vi "PI-C867-Joystick.vi"() -> ()   [LabVIEW 2026]
doc: "Demonstrates the fundamentals of the State Machine design pattern in LabVIEW. A state machine, in its simplest form, is a case structure within a while loop, with a state enum wired to a shift register on the loop to define the execution of different cases (or \"states\") of the case structure on different iterations of the loop."
uses:
  States.ctl
panel:
  out "WAIT":bool
  out "JoystickID":i32=3
  out "C687 Axes":string[](array[string])
  out "C687 System No.":i32=2
  out "Current positions":dbl[](array[numeric])=[0.0, -0.0002] format="%.6f"
  in  "Velocity array":dbl[](array[numeric])=[0.05, 0.1, 0.25, 0.5, 1.0, 10.0]
  in  "Joystick":bool
  out "Current velocity":dbl[](array[numeric])=[10.0, 10.0] format="%.6f"
  in  "Stop":bool
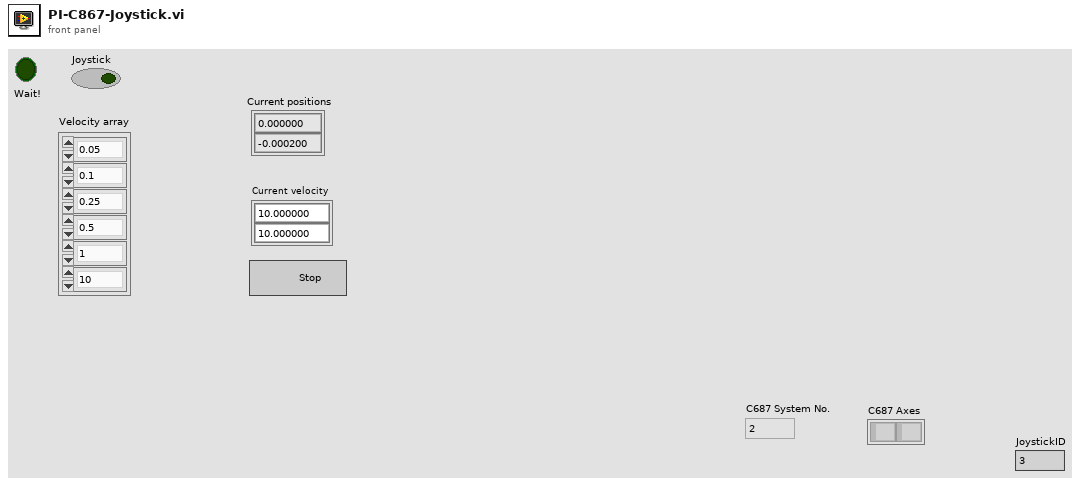
[diagram p1: front panel]
types:
  T1 = typedef "States.ctl" = enum16{"Initialize", "Wait for Event", "Joystick ON/OFF", "Button Pressed", "Stop"}
  T2 = cluster{"C687 System No.":i32, "JoystickID to query":i32[], "Conn.  Axes":string[], "State":bool[][], "Current velocity":dbl[], "Current positions":dbl[]}
  T3 = cluster{"RON Affected axes":string[], "Reference mode":bool[], "Check FRF?":bool}
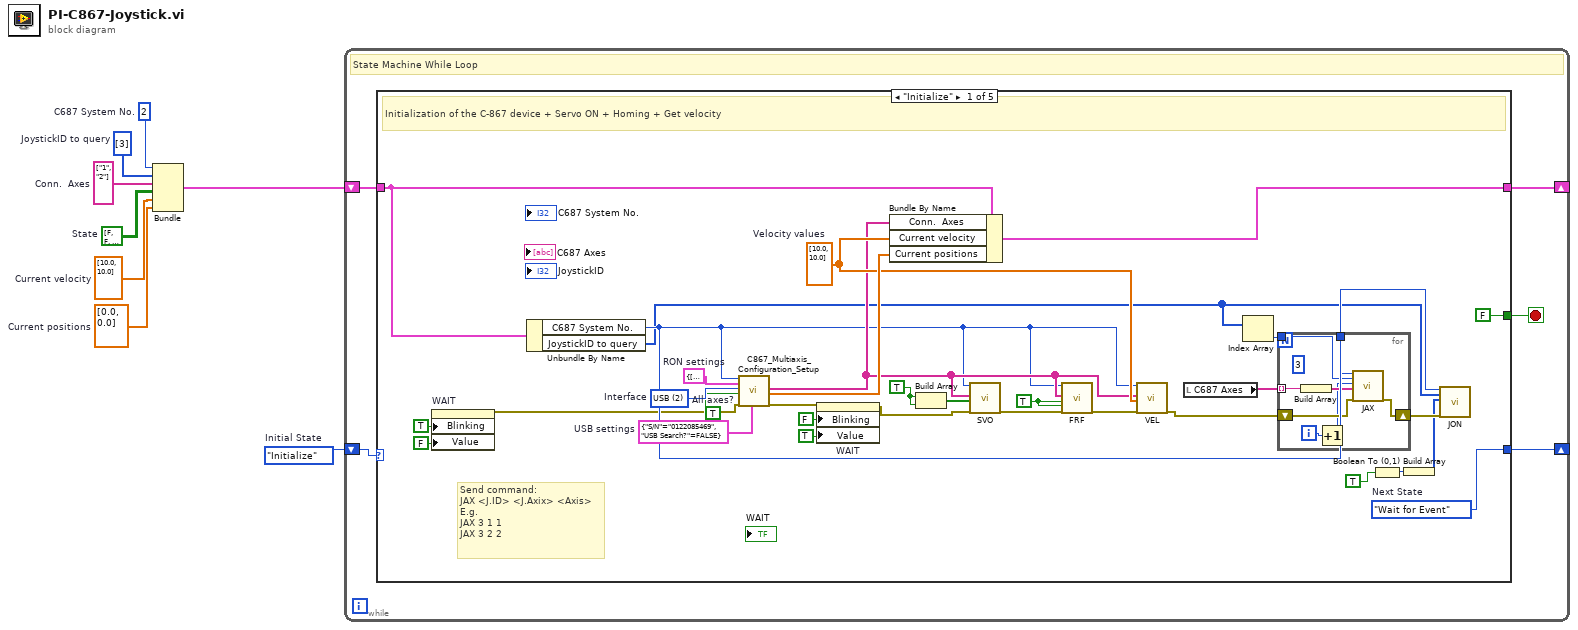
[diagram p0: block diagram]
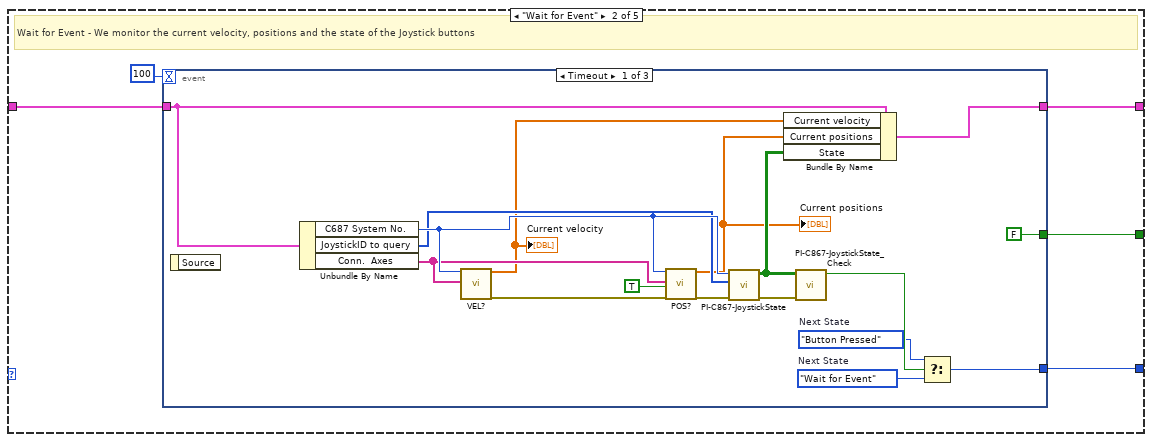
[diagram p2: hidden frame]
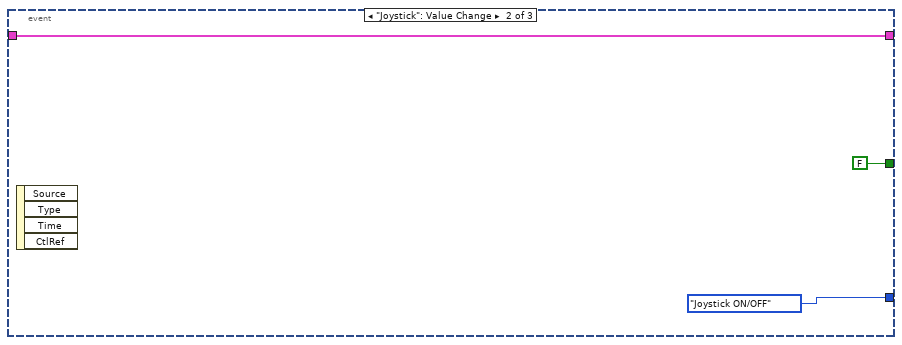
[diagram p3: hidden frame]
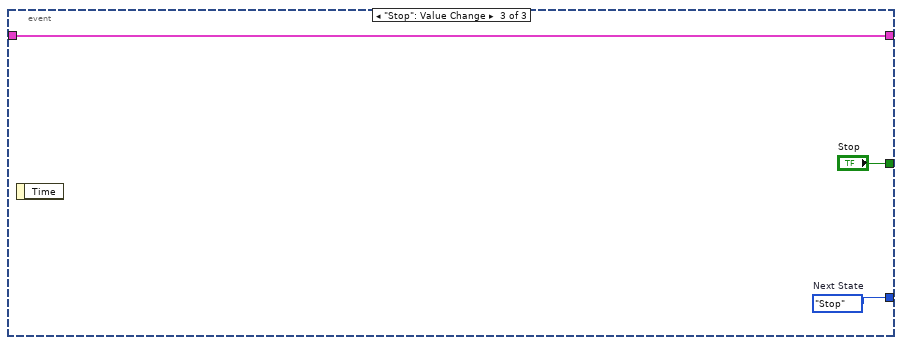
[diagram p4: hidden frame]
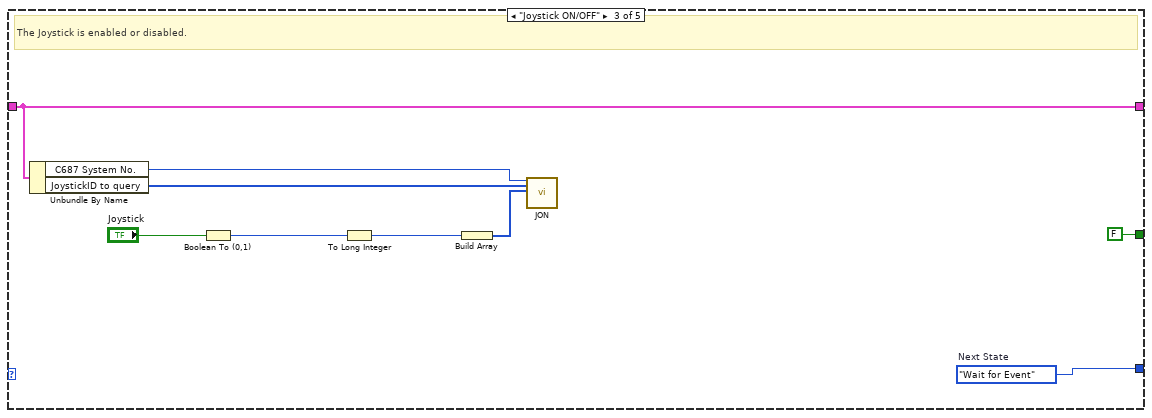
[diagram p5: hidden frame]
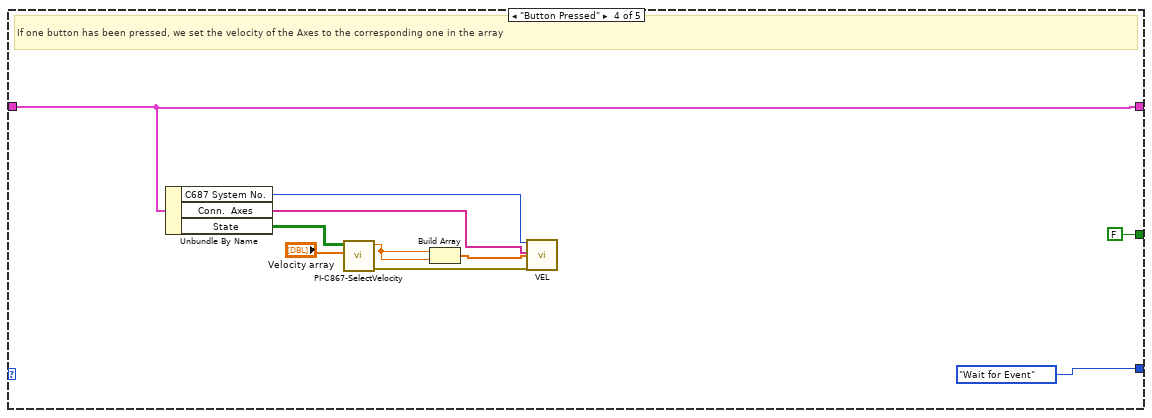
[diagram p6: hidden frame]
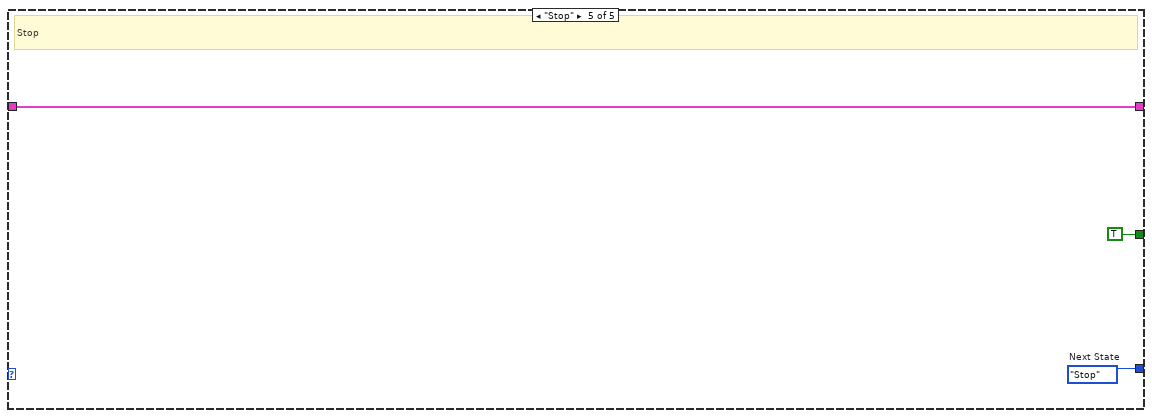
[diagram p7: hidden frame]
diagram:
  w1 = dbl[] [0.0, 0.0]  # Current positions
  w2 = dbl[] [10.0, 10.0]  # Current velocity
  w4 = bool[][] [[FALSE], [FALSE], [FALSE], [FALSE], [FALSE], [FALSE]]  # State
  w5 = string[] ["1", "2"]  # Conn.  Axes
  w6 = i32[] [3]  # JoystickID to query
  w7 = 2  # C687 System No.
  w8 = States."Initialize"  # Initial State
  n1 = Bundle("C687 System No."=w7, "JoystickID to query"=w6, "Conn.  Axes"=w5, "State"=w4, "Current velocity"=w2, "Current positions"=w1) -> (w3:T2)  [unwired: 1 in]
  n2 = while {
    shift-right: [w12] -> _
    shift-left: w8 -> [w13]
    shift-right: [w9] -> _
    shift-left: w3 -> [w10]
    stop <- w11 stop-if-true
    # "State Machine While Loop"
    n3 = case "State Machine Case Structure" shown="\"Initialize\"" w13 {
      tunnel: [w45 w58 w90 States."Wait for Event" ("(Value Not Used)") w103] -> w12
      tunnel: [FALSE ("Stop the Loop") w57 FALSE ("Stop the Loop") FALSE ("Stop the Loop") TRUE ("Stop the Loop")] -> w11
      tunnel: w10 -> [w35 w55 w84 w94 w101]
      tunnel: [w33 w54 w84 w94 w101] -> w9
      frame "Initialize" {
        w32 = dbl[] [10.0, 10.0]  # Velocity values
        w30 = TRUE ("Axis identifier?")
        w39 = TRUE ("Switch Servo on")
        w40 = T3 {"RON Affected axes"=[], "Reference mode"=[], "Check FRF?"=TRUE}  # RON settings
        w43 = u16 2 items=["RS232", "RS232 DaisyChain", "USB", "USB DaisyChain"]  # Interface
        w42 = cluster{"S/N":string, "USB Search?":bool} {"S/N"="0122085469", "USB Search?"=FALSE}  # USB settings
        w41 = TRUE  # All axes?
        w45 = States."Wait for Event"  # Next State
        # "Send command:\nJAX <J.ID> <J.Axix> <Axis>\nE.g.\nJAX 3 1 1\nJAX 3 2 2"
        # "Initialization of the C-867 device + Servo ON + Homing + Get velocity"
        n4 = property on="WAIT" class="Bool (strict)"("Blinking"=TRUE, "Value"=FALSE ("WAIT")) -> (error out=w18:errorcluster)  [unwired: 2 in, 1 out]
        n5 = Unbundle By Name(w35) -> ("C687 System No."=w27:i32, "JoystickID to query"=w22:i32[])
        n6 = call "C867_Multiaxis_Configuration_Setup.vi"("System no."=w27, "RON settings"=w40, "Interface"=w43, "All axes?"=w41, "error in"=w18, "USB settings"=w42) -> ("Conn. \nAxes"=w31:string[], "Position"=w34:dbl[], "error out"=w15:errorcluster)  [unwired: 7 in, 4 out]
        n7 = property on="WAIT" class="Bool (strict)"(error in=w15, "Blinking"=FALSE, "Value"=TRUE ("WAIT")) -> (error out=w14:errorcluster)  [unwired: 1 in, 1 out]
        n8 = Bundle By Name(cluster=w35, "Conn.  Axes"=w31, "Current velocity"=w32, "Current positions"=w34) -> (w33:T2)
        n9 = Build Array(w39, w39) -> (w38:bool[])
        n10 = call "SVO.vi"("System no."=w27, "Axes to command"=w31, "Servo mode"=w38, "error in"=w14) -> ("error out"=w37:errorcluster)  [unwired: 15 in]
        n11 = call "FRF.vi"("System no."=w27, "Affected axes"=w31, "All axes?"=w30, "Axis identifier?"=w30, "error in"=w37) -> ("error out"=w36:errorcluster)  [unwired: 14 in]
        n12 = call "VEL.vi"("System no."=w27, "Axes to set"=w31, "Velocity values"=w32, "error in"=w36) -> ("error out"=w26:errorcluster)  [unwired: 14 in, 1 out]
        n13 = local read "C687 Axes"() -> (w29:string[])
        n14 = Index Array(array=w22) -> (element=w21:i32)  [unwired: 1 in]
        n15 = for {
          tunnel: w27 -> [w48]
          tunnel: w29 -> [w52] mode=indexing
          shift-right: [w47] -> w28
          shift-left: w26 -> [w53]
          tunnel: w21 -> [w46]
          i -> [w50]
          (unwired) 3 ("JoystickID")
          n16 = Build Array(w52) -> (w51:string[])
          n17 = Increment(x=w50) -> (x+1=w49:i32)
          n18 = call "JAX.vi"("System no."=w48, "JoystickID"=w46, "Joystick axis"=w49, "Axes to set"=w51, "error in"=w53) -> ("error out"=w47:errorcluster)  [unwired: 14 in]
        }
        n19 = Boolean To (0,1)(Boolean=TRUE) -> (0, 1=w25:i16)
        n20 = Build Array(w25) -> (w23:i16[])
        n21 = call "JON.vi"("System no."=w27, "JoystickID to set"=w22, "Joystick mode"=w23, "error in"=w28) -> ()  [unwired: 14 in, 2 out]
      }
      frame "Wait for Event" {
        # "Wait for Event - We monitor the current velocity, positions and the state of the Joystick buttons"
        n22 = event shown="[0] Timeout" {
          selector: _ -> [_ _ _]
          dyn-events: _ -> [_ _ _]
          timeout: 100 -> [_ _ _]
          tunnel: [w70 States."Joystick ON/OFF" ("Next State") w81] -> w58
          tunnel: [FALSE ("Stop") FALSE ("Stop") "Stop"] -> w57
          tunnel: w55 -> [w62 w76 w79]
          tunnel: [w63 w76 w79] -> w54
          event Timeout {
            w67 = States."Button Pressed"  # Next State
            w68 = States."Wait for Event"  # Next State
            n23 = event-data() -> ()  [unwired: 1 in, 1 out]
            n24 = Unbundle By Name(w62) -> ("C687 System No."=w66:i32, "JoystickID to query"=w65:i32[], "Conn.  Axes"=w64:string[])
            n25 = call "VEL?.vi"("System no."=w66, "Axes to query"=w64) -> ("Velocity"=w59:dbl[], "error out"=w74:errorcluster)  [unwired: 16 in]
            "Current velocity" <- w59
            n26 = call "POS?.vi"("System no."=w66, "Axes to query"=w64, "All axes?"=TRUE, "error in"=w74) -> ("Position"=w60:dbl[], "error out"=w72:errorcluster)  [unwired: 14 in]
            "Current positions" <- w60
            n27 = call "PI-C867-JoystickState.vi"("error in"=w72, "JoystickID to query"=w65, "System no."=w66) -> ("error out"=w71:errorcluster, "State"=w61:bool[][])  [unwired: 7 in]
            n28 = Bundle By Name(cluster=w62, "Current velocity"=w59, "Current positions"=w60, "State"=w61) -> (w63:T2)
            n29 = call "PI-C867-JoystickState_Check.vi"("error in (no error)"=w71, "State in"=w61) -> ("All 0?"=w69:bool)  [unwired: 8 in, 1 out]
            n30 = Select(t=w67, s=w69, f=w68) -> (s? t:f=w70:T1)
          }
          event "Joystick": Value Change {
            n31 = event-data() -> ()  [unwired: 1 in, 4 out]
          }
          event "Stop": Value Change {
            w81 = States."Stop"  # Next State
            n32 = event-data() -> ()  [unwired: 1 in, 1 out]
          }
        }
      }
      frame "Joystick ON/OFF" {
        w90 = States."Wait for Event"  # Next State
        # "The Joystick is enabled or disabled."
        n33 = Unbundle By Name(w84) -> ("C687 System No."=w83:i32, "JoystickID to query"=w82:i32[])
        n34 = Boolean To (0,1)(Boolean="Joystick") -> (0, 1=w85:i16)
        n35 = To Long Integer(number=w85) -> (32bit integer=w86:i32)
        n36 = Build Array(w86) -> (w88:i32[])
        n37 = call "JON.vi"("System no."=w83, "JoystickID to set"=w82, "Joystick mode"=w88) -> ()  [unwired: 15 in, 2 out]
      }
      frame "Button Pressed" {
        # "If one button has been pressed, we set the velocity of the Axes to the corresponding one in the array"
        n38 = Unbundle By Name(w94) -> ("C687 System No."=w93:i32, "Conn.  Axes"=w92:string[], "State"=w91:bool[][])
        n39 = call "PI-C867-SelectVelocity.vi"("Velocity array"="Velocity array", "State"=w91) -> ("error out"=w97:errorcluster, "Velocity out"=w96:dbl)  [unwired: 8 in]
        n40 = Build Array(w96, w96) -> (w95:dbl[])
        n41 = call "VEL.vi"("System no."=w93, "Axes to set"=w92, "Velocity values"=w95, "error in"=w97) -> ()  [unwired: 14 in, 2 out]
      }
      frame "Stop" {
        w103 = States."Stop"  # Next State
        # "Stop"
      }
    }
  }
